vi "CCD photon image_Shaowei-v2.vi"() -> ()   [LabVIEW 2009]
uses:
  <vilib>/Utility/file.llb/Read From Spreadsheet File (DBL).vi
  Instance           5 35Saved   CCD photon image_540_800_CR .vi
  Instance           4 35Saved   CCD photon image_540_800_CR .vi
  Instance           3 35Saved   CCD photon image_540_800_CR .vi
  Instance           8 35Saved   CCD photon image_540_800_CR .vi
  <vilib>/Analysis/Matrix/Numeric/Conversions/Array To Matrix - RA2.vi
  Instance          12 35Saved   CCD photon image_540_800_CR .vi
  Instance          18 35Saved   CCD photon image_540_800_CR .vi
  <vilib>/Analysis/Matrix/NI_Matrix.lvlib
panel:
  in  "Save Matrix6":bool
  in  "Save Matrix5":bool
  in  "Save Matrix3":bool
  in  "Save Matrix4":bool
  out "Matrix 2":string
  in  "Save Matrix2":bool
  out "Matrix 1":string
  in  "Save Matrix1":bool
  in  "select 2":bool
  in  "select":bool
  in  "next 2":bool
  in  "next":bool
  in  "previous 2":bool
  in  "previous":bool
  in  "?":bool
  out "?":path
  out "?":path
  out "?":i32
  in  "?":bool
  in  "stop 2":bool
  in  "#6":bool
  in  "#5":bool
  in  "to":dbl=950.0
  in  "From":dbl=550.0
  out "Intensity Graph 6":dbl[][](graph)
  out "Col":dbl
  out "to":dbl
  out "Matrix 6":string
  in  "lstart (nm)":dbl
  in  "lend (nm)":dbl
  out "eV":dbl
  out "eV":dbl
  out "Intensity Graph 5":dbl[][](graph)
  out "Col":dbl
  out "to":dbl
  out "Matrix 5":string
  in  "lstart (nm)":dbl
  in  "lend (nm)":dbl
  out "eV":dbl
  out "eV":dbl
  in  "?":bool
  out "MAX":dbl
  out "MIN":dbl
  out "X":sgl
  out "Y":sgl
  out "to":dbl
  out "Col":dbl
  out "eV":dbl
  out "eV":dbl
  in  "lend (nm)":dbl
  in  "lstart (nm)":dbl
  out "eV":dbl
  out "eV":dbl
  in  "lend (nm)":dbl
  in  "lstart (nm)":dbl
  out "to":dbl
  out "Col":dbl
  out "to":dbl
  out "Col":dbl
  out "eV":dbl
  out "eV":dbl
  in  "lend (nm)":dbl
  in  "lstart (nm)":dbl
  in  "?":dbl=32.0
  out "eV":dbl
  out "eV":dbl
  in  "lend (nm)":dbl
  in  "lstart (nm)":dbl
  out "to":dbl
  out "Col":dbl
  in  "#3":bool
  in  "#4":bool
  in  "#2":bool
  out "Intensity Graph 4":dbl[][](graph)
  out "Matrix 4":string
  out "Intensity Graph 3":dbl[][](graph)
  out "Matrix 3":string
  out "Intensity Graph 2":dbl[][](graph)
  out "Intensity Graph":dbl[][](graph)
  # "Input File"
  # "2 Files"
  # "1 File"
  # "1st"
  # "2nd"
  # "Spectra Range"
  # "nm"
  # "nm"
  # "# of Pixel"
  # "Image Size"
  # "Bit"
  # "Active Matrix"
  # "ON"
  # "OFF"
  # "Cosmic Ray Removal"
  # "NO"
  # "YES"
  # "Value"
  # "Position"
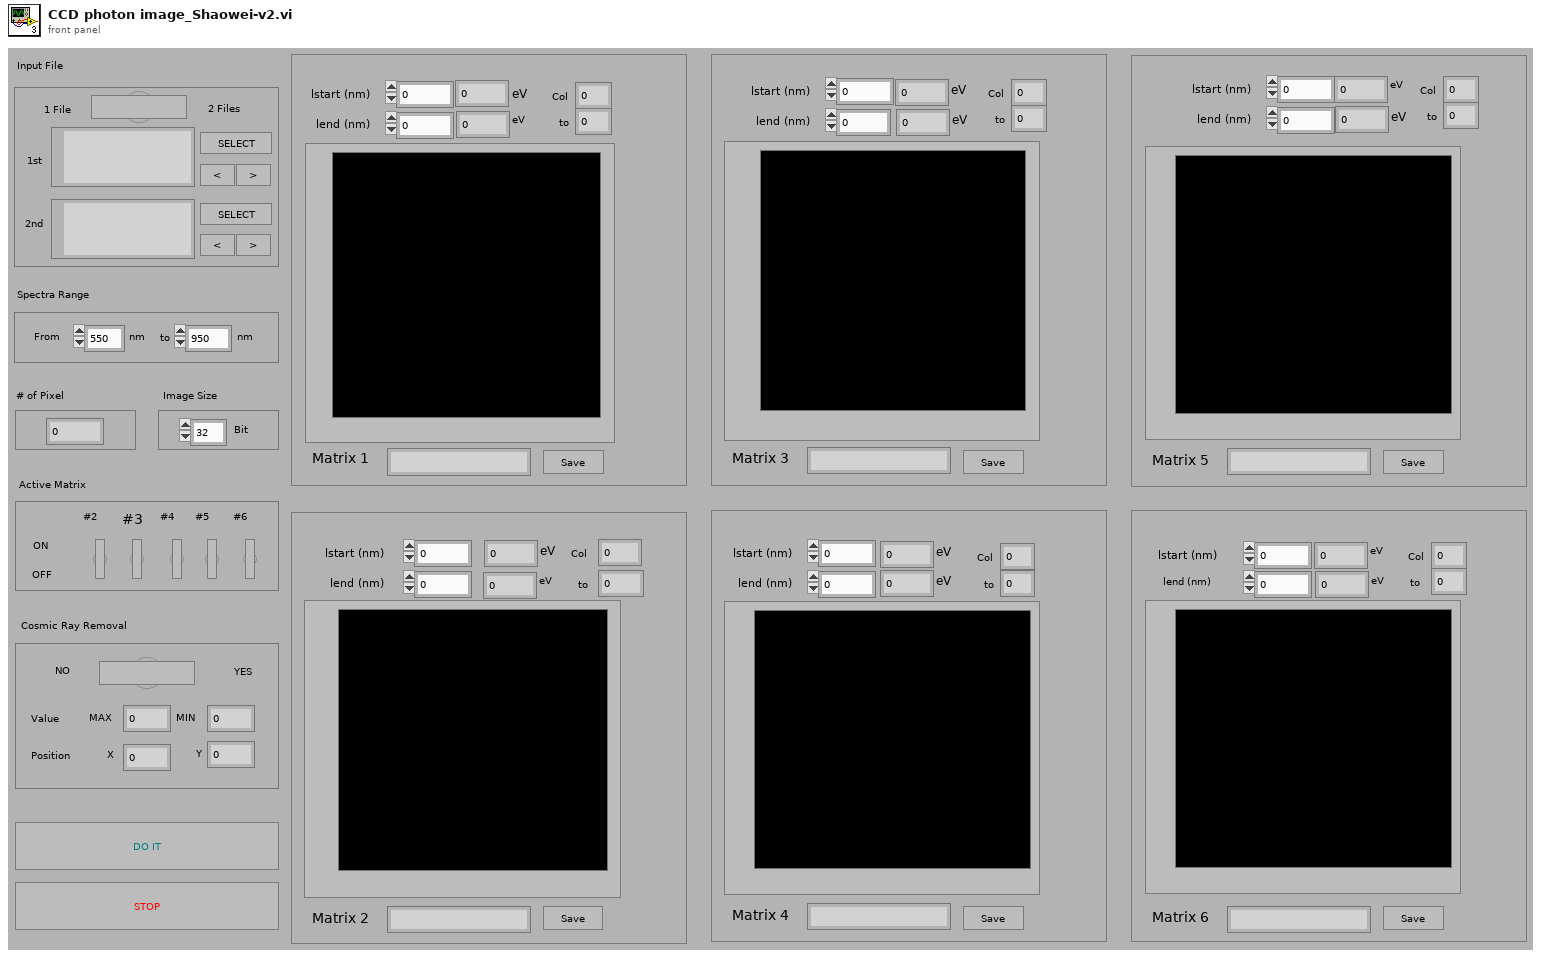
[diagram p1: front panel]
types:
  T1 = typedef "NI_Matrix.lvlib/RealMatrix.ctl" = dbl[][]
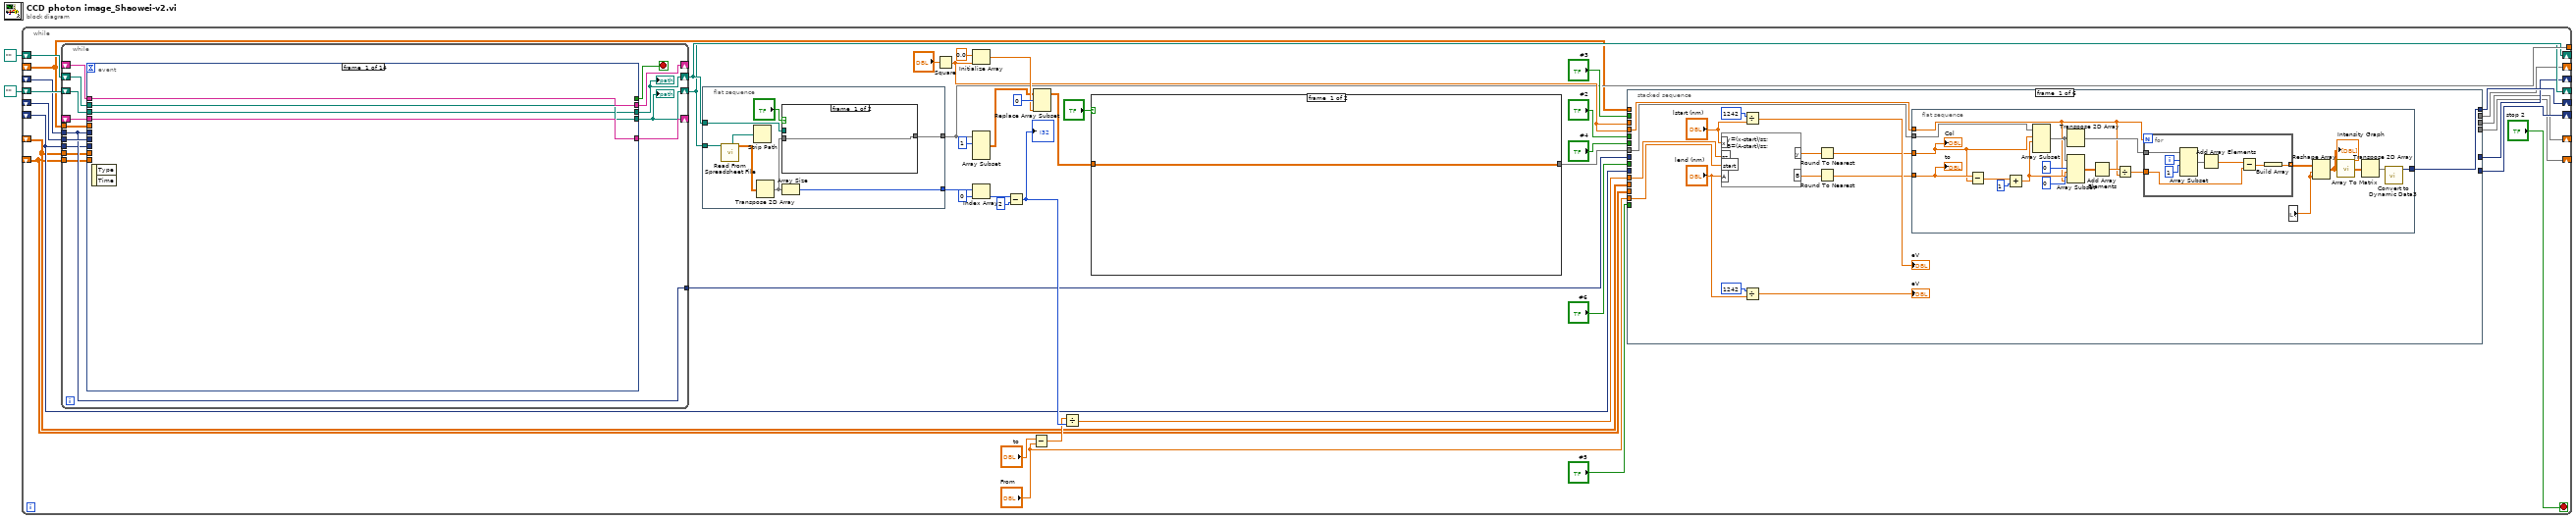
[diagram p0: block diagram]
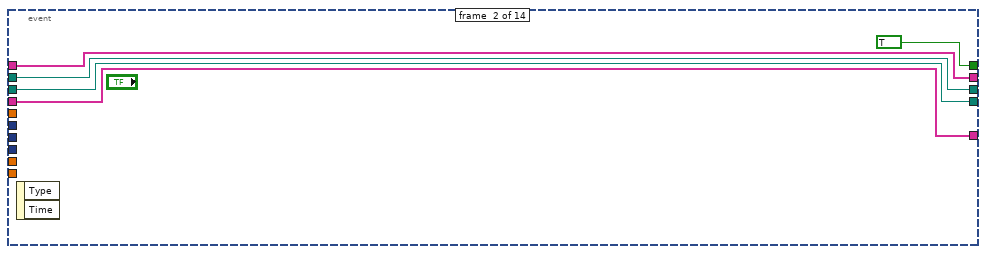
[diagram p2: hidden frame]
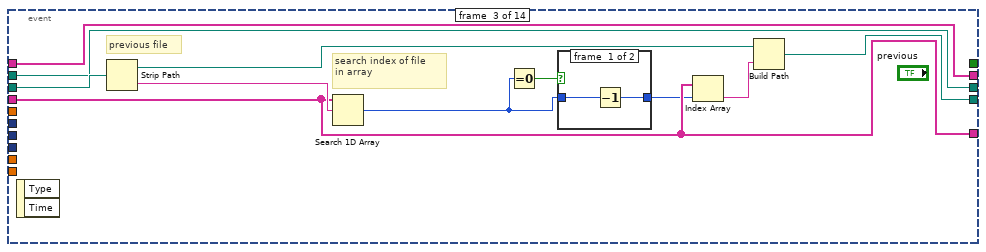
[diagram p3: hidden frame]
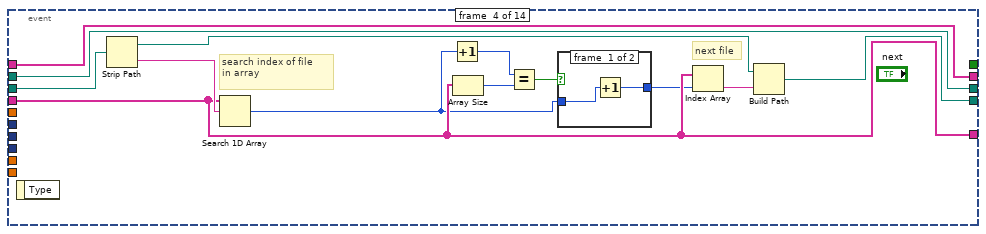
[diagram p5: hidden frame]
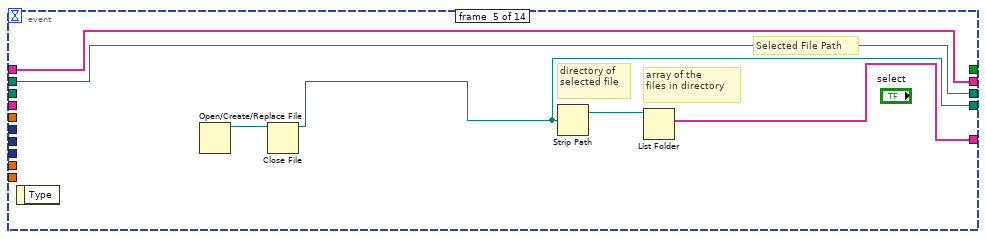
[diagram p7: hidden frame]
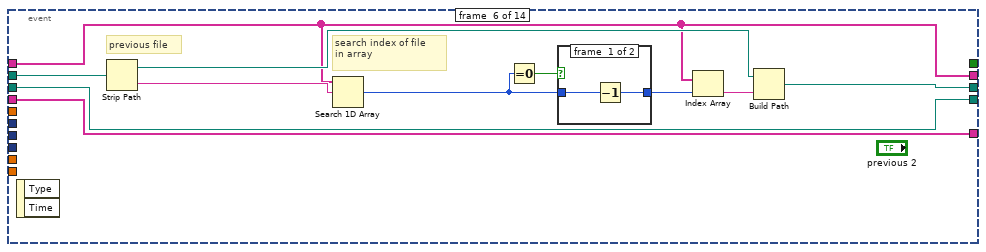
[diagram p8: hidden frame]
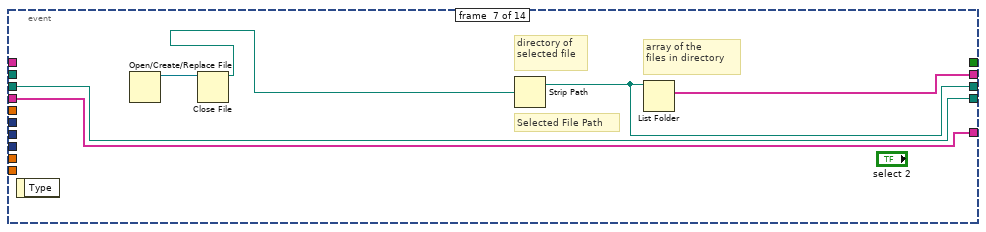
[diagram p10: hidden frame]
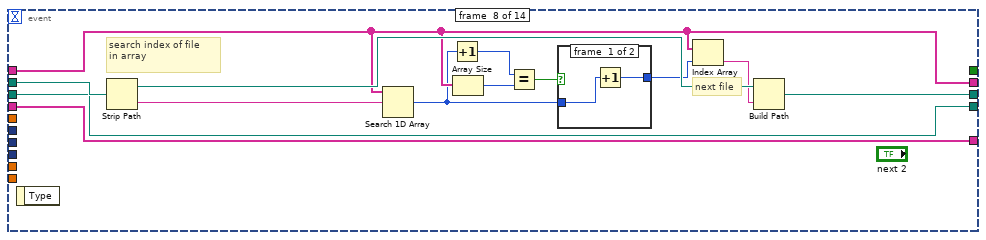
[diagram p11: hidden frame]
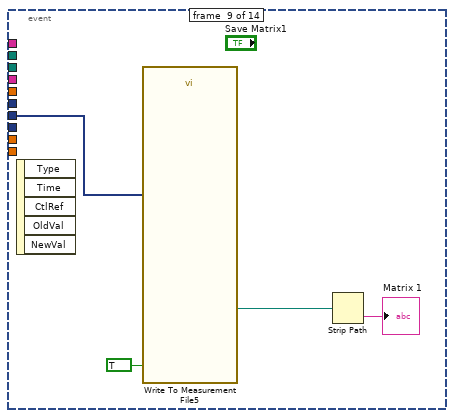
[diagram p13: hidden frame]
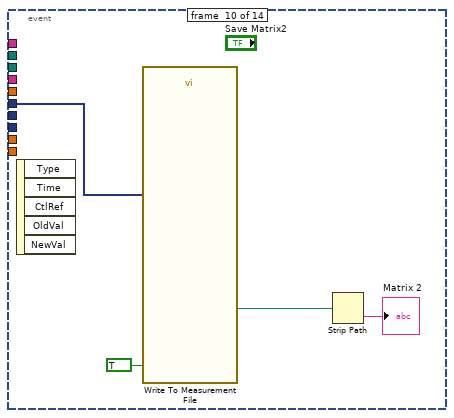
[diagram p14: hidden frame]
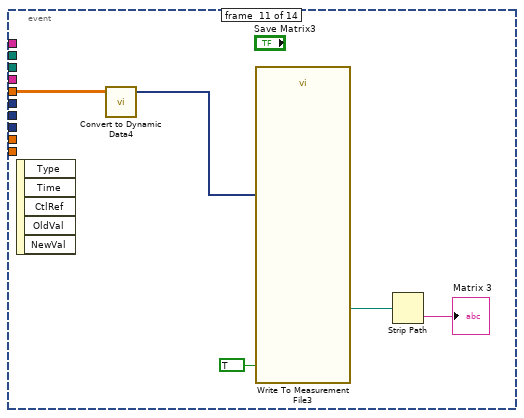
[diagram p15: hidden frame]
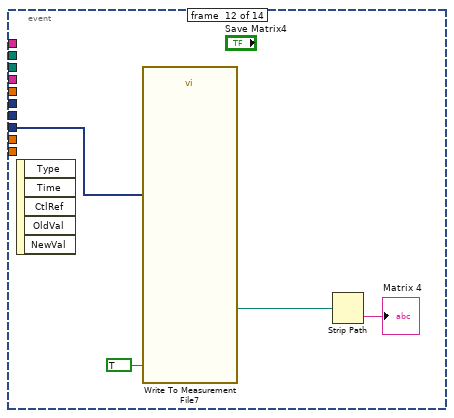
[diagram p16: hidden frame]
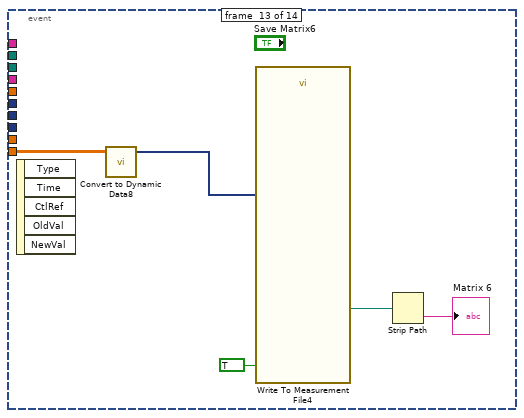
[diagram p17: hidden frame]
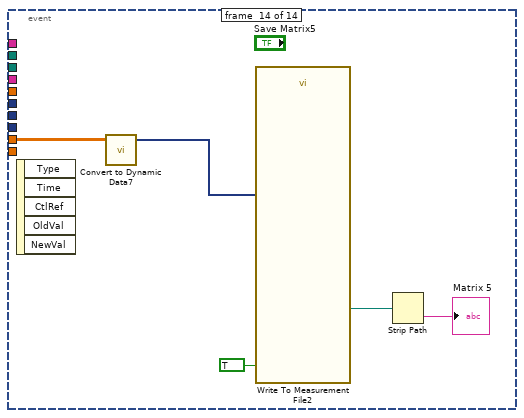
[diagram p18: hidden frame]
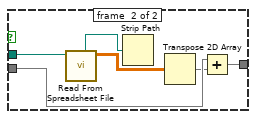
[diagram p19: hidden frame]
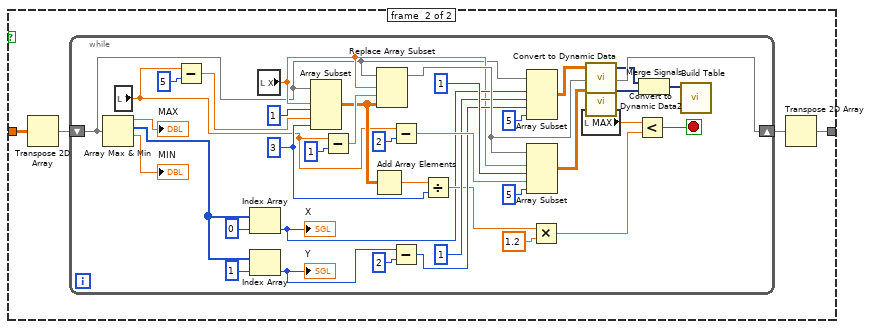
[diagram p20: hidden frame]
diagram:
  n1 = while {
    tunnel: [w26] -> _
    shift-right: [w16] -> _
    shift-left: path "" ("path") -> [w18]
    shift-right: [w17] -> _
    shift-left: path "" ("path") -> [w19]
    shift-right: [w15] -> _
    shift-left: _ -> [w14]
    shift-right: [w13] -> _
    shift-left: _ -> [w12]
    shift-right: [w10] -> _
    shift-left: _ -> [w9]
    shift-right: [w8] -> _
    shift-left: _ -> [w7]
    shift-right: [w6] -> _
    shift-left: _ -> [w5]
    shift-right: [w4] -> _
    shift-left: _ -> [w3]
    stop <- "stop 2" stop-if-true
    n2 = while {
      shift-right: [w60] -> _
      shift-left: _ -> [w59]
      shift-right: [w46] -> w16
      shift-left: w18 -> [w58]
      shift-right: [w47] -> w17
      shift-left: w19 -> [w57]
      shift-right: [w56] -> _
      shift-left: _ -> [w55]
      tunnel: w14 -> [w53]
      tunnel: w12 -> [w52]
      tunnel: [w52] -> w11
      tunnel: w9 -> [w51]
      tunnel: w7 -> [w50]
      tunnel: w5 -> [w49]
      tunnel: w3 -> [w48]
      stop <- w54 stop-if-true
      n3 = event shown="[4] \"select\": Value Change" {
        selector: _ -> [_ _ _ _ _ _ _ _ _ _ _ _ _ _]
        dyn-events: _ -> [_ _ _ _ _ _ _ _ _ _ _ _ _ _]
        timeout: _ -> [_ _ _ _ _ _ _ _ _ _ _ _ _ _]
        tunnel: [_ TRUE _ _ _ _ _ _ _ _ _ _ _ _] -> w54
        tunnel: [w63 w67 w75 w93 w100 w106 w124 w133 _ _ _ _ _ _] -> w46
        tunnel: [w64 w68 w77 w89 w104 w111 w123 w132 _ _ _ _ _ _] -> w60
        tunnel: w59 -> [w64 w68 w77 w89 _ w111 w123 w132 _ _ _ _ _ _]
        tunnel: w58 -> [w63 w67 w80 w92 _ w106 w124 w133 _ _ _ _ _ _]
        tunnel: [w61 w65 w73 w90 w102 w107 w122 w134 _ _ _ _ _ _] -> w47
        tunnel: w57 -> [w61 w65 w73 w90 w102 w113 _ w135 _ _ _ _ _ _]
        tunnel: [w62 w66 w74 w91 w103 w112 w125 w128 _ _ _ _ _ _] -> w56
        tunnel: w55 -> [w62 w66 w74 w91 w103 w112 _ w128 _ _ _ _ _ _]
        tunnel: w53 -> [_ _ _ _ _ _ _ _ w145 _ _ _ _ _]
        tunnel: w52 -> [_ _ _ _ _ _ _ _ _ w149 _ _ _ _]
        tunnel: w51 -> [_ _ _ _ _ _ _ _ _ _ _ w155 _ _]
        tunnel: w50 -> [_ _ _ _ _ _ _ _ _ _ w151 _ _ _]
        tunnel: w49 -> [_ _ _ _ _ _ _ _ _ _ _ _ _ w166]
        tunnel: w48 -> [_ _ _ _ _ _ _ _ _ _ _ _ w160 _]
        event #0 {
          n4 = event-data() -> ()  [unwired: 1 in, 2 out]
        }
        event #1 {
          n5 = event-data() -> ()  [unwired: 1 in, 2 out]
        }
        event #2 {
          # "previous file"
          # "search index of file\nin array"
          n6 = event-data() -> ()  [unwired: 1 in, 2 out]
          n7 = Strip Path(path=w80) -> (stripped path=w78:path, name=w79:string)
          n8 = Search 1D Array(1D array=w77, element=w79) -> (index of element=w71:i32)  [unwired: 1 in]
          n9 = Equal To 0?(x=w71) -> (x = 0?=w72:bool)
          n10 = case shown="False" w72 {
            tunnel: w71 -> [w82 w83]
            tunnel: [w81 w83] -> w70
            frame #0 {
              n11 = Decrement(x=w82) -> (x-1=w81:i32)
            }
            frame #1 {
            }
          }
          n12 = Index Array(array=w77, index=w70) -> (element=w76:string)
          n13 = Build Path(base path=w78, name or relative path=w76) -> (appended path=w75:path)
        }
        event #3 {
          # "next file"
          # "search index of file\nin array"
          n14 = event-data() -> ()  [unwired: 1 in, 1 out]
          n15 = Strip Path(path=w92) -> (stripped path=w95:path, name=w96:string)
          n16 = Search 1D Array(1D array=w89, element=w96) -> (index of element=w84:i32)  [unwired: 1 in]
          n17 = Increment(x=w84) -> (x+1=w85:i32)
          n18 = Array Size(array=w89) -> (size(s)=w88:i32)
          n19 = Equal?(x=w85, y=w88) -> (x = y?=w87:bool)
          n20 = case shown="True" w87 {
            tunnel: w84 -> [w98 w99]
            tunnel: [w97 w99] -> w86
            frame #0 {
              n21 = Increment(x=w98) -> (x+1=w97:i32)
            }
            frame #1 {
            }
          }
          n22 = Index Array(array=w89, index=w86) -> (element=w94:string)
          n23 = Build Path(base path=w95, name or relative path=w94) -> (appended path=w93:path)
        }
        event #4 {
          # "array of the \nfiles in directory"
          # "directory of\nselected file"
          # "Selected File Path"
          n24 = event-data() -> ()  [unwired: 1 in, 1 out]
          n25 = Open/Create/Replace File() -> (refnum out=w101:refnum<file>)  [unwired: 6 in, 2 out]
          n26 = Close File(refnum=w101) -> (path=w100:path)  [unwired: 1 in, 1 out]
          n27 = Strip Path(path=w100) -> (stripped path=w105:path)  [unwired: 1 out]
          n28 = List Folder(path=w105) -> (filenames=w104:string[])  [unwired: 3 in, 3 out]
        }
        event #5 {
          # "previous file"
          # "search index of file\nin array"
          n29 = event-data() -> ()  [unwired: 1 in, 2 out]
          n30 = Strip Path(path=w113) -> (stripped path=w115:path, name=w116:string)
          n31 = Search 1D Array(1D array=w112, element=w116) -> (index of element=w109:i32)  [unwired: 1 in]
          n32 = Equal To 0?(x=w109) -> (x = 0?=w110:bool)
          n33 = case shown="False" w110 {
            tunnel: w109 -> [w118 w119]
            tunnel: [w117 w119] -> w108
            frame #0 {
              n34 = Decrement(x=w118) -> (x-1=w117:i32)
            }
            frame #1 {
            }
          }
          n35 = Index Array(array=w112, index=w108) -> (element=w114:string)
          n36 = Build Path(base path=w115, name or relative path=w114) -> (appended path=w107:path)
        }
        event #6 {
          # "array of the \nfiles in directory"
          # "directory of\nselected file"
          # "Selected File Path"
          n37 = event-data() -> ()  [unwired: 1 in, 1 out]
          n38 = Open/Create/Replace File() -> (refnum out=w121:refnum<file>)  [unwired: 6 in, 2 out]
          n39 = Close File(refnum=w121) -> (path=w120:path)  [unwired: 1 in, 1 out]
          n40 = Strip Path(path=w120) -> (stripped path=w122:path)  [unwired: 1 out]
          n41 = List Folder(path=w122) -> (filenames=w125:string[])  [unwired: 3 in, 3 out]
        }
        event #7 {
          # "next file"
          # "search index of file\nin array"
          n42 = event-data() -> ()  [unwired: 1 in, 1 out]
          n43 = Strip Path(path=w135) -> (stripped path=w137:path, name=w138:string)
          n44 = Search 1D Array(1D array=w128, element=w138) -> (index of element=w127:i32)  [unwired: 1 in]
          n45 = Increment(x=w127) -> (x+1=w129:i32)
          n46 = Array Size(array=w128) -> (size(s)=w131:i32)
          n47 = Equal?(x=w129, y=w131) -> (x = y?=w130:bool)
          n48 = case shown="True" w130 {
            tunnel: w127 -> [w140 w141]
            tunnel: [w139 w141] -> w126
            frame #0 {
              n49 = Increment(x=w140) -> (x+1=w139:i32)
            }
            frame #1 {
            }
          }
          n50 = Index Array(array=w128, index=w126) -> (element=w136:string)
          n51 = Build Path(base path=w137, name or relative path=w136) -> (appended path=w134:path)
        }
        event #8 {
          n52 = event-data() -> ()  [unwired: 1 in, 5 out]
          n53 = call "Write To Measurement File5"("Signals"=w145, "Reset"=TRUE) -> ("Filename Out"=w143:path)  [unwired: 15 in, 2 out]
          n54 = Strip Path(path=w143) -> (name=→"Matrix 1":string)  [unwired: 1 out]
        }
        event #9 {
          n55 = event-data() -> ()  [unwired: 1 in, 5 out]
          n56 = call "Write To Measurement File"("Signals"=w149, "Reset"=TRUE) -> ("Filename Out"=w147:path)  [unwired: 15 in, 2 out]
          n57 = Strip Path(path=w147) -> (name=→"Matrix 2":string)  [unwired: 1 out]
        }
        event #10 {
          n58 = event-data() -> ()  [unwired: 1 in, 5 out]
          n59 = call "Convert to Dynamic Data4"("2D Array"=w151) -> ("Dynamic Data Type"=w150:dynamicdata)  [unwired: 3 in]
          n60 = call "Write To Measurement File3"("Signals"=w150, "Reset"=TRUE) -> ("Filename Out"=w154:path)  [unwired: 15 in, 2 out]
          n61 = Strip Path(path=w154) -> (name=→"Matrix 3":string)  [unwired: 1 out]
        }
        event #11 {
          n62 = event-data() -> ()  [unwired: 1 in, 5 out]
          n63 = call "Write To Measurement File7"("Signals"=w155, "Reset"=TRUE) -> ("Filename Out"=w157:path)  [unwired: 15 in, 2 out]
          n64 = Strip Path(path=w157) -> (name=→"Matrix 4":string)  [unwired: 1 out]
        }
        event #12 {
          n65 = event-data() -> ()  [unwired: 1 in, 5 out]
          n66 = call "Convert to Dynamic Data8"("2D Array"=w160) -> ("Dynamic Data Type"=w159:dynamicdata)  [unwired: 3 in]
          n67 = call "Write To Measurement File4"("Signals"=w159, "Reset"=TRUE) -> ("Filename Out"=w162:path)  [unwired: 15 in, 2 out]
          n68 = Strip Path(path=w162) -> (name=→"Matrix 6":string)  [unwired: 1 out]
        }
        event #13 {
          n69 = event-data() -> ()  [unwired: 1 in, 5 out]
          n70 = call "Convert to Dynamic Data7"("2D Array"=w166) -> ("Dynamic Data Type"=w165:dynamicdata)  [unwired: 3 in]
          n71 = call "Write To Measurement File2"("Signals"=w165, "Reset"=TRUE) -> ("Filename Out"=w167:path)  [unwired: 15 in, 2 out]
          n72 = Strip Path(path=w167) -> (name=→"Matrix 5":string)  [unwired: 1 out]
        }
      }
      "?" <- w46
      "?" <- w47
    }
    n73 = flat-sequence {
      tunnel: [w175] -> w26
      tunnel: [w172] -> w23
      tunnel: w16 -> [w170]
      tunnel: w17 -> [w169]
      frame #0 {
        n74 = call-poly <vilib>:"Read From Spreadsheet File.vi"("file path (dialog if empty)"=w170) -> ("all rows"=w173:dbl[][], "new file path (Not A Path if cancelled)"=w176:path)  [unwired: 6 in, 3 out]
        n75 = Strip Path(path=w176) -> ()  [unwired: 2 out]
        n76 = Transpose 2D Array(2D array=w173) -> (transposed array=w171:dbl[][])
        n77 = case shown="False" "?" {
          tunnel: w171 -> [w177 w182]
          tunnel: [w177 w181] -> w175
          tunnel: w169 -> [_ w178]
          frame #0 {
          }
          frame #1 {
            n78 = call-poly <vilib>:"Read From Spreadsheet File.vi"("file path (dialog if empty)"=w178) -> ("all rows"=w180:dbl[][], "new file path (Not A Path if cancelled)"=w183:path)  [unwired: 6 in, 3 out]
            n79 = Strip Path(path=w183) -> ()  [unwired: 2 out]
            n80 = Transpose 2D Array(2D array=w180) -> (transposed array=w179:dbl[][])
            n81 = Add(x=w182, y=w179) -> (x+y=w181:dbl[][])
          }
        }
        n82 = Array Size(array=w171) -> (size(s)=w172:i32[])
      }
    }
    n83 = Square(x="?") -> (x^2=w37:dbl)
    n84 = Initialize Array(0.0 ("element"), w37) -> (w41:dbl[])
    n85 = Array Subset(array=w26, index (row)=1) -> (w39:dbl[][])  [unwired: 3 in]
    n86 = Index Array(array=w23, index=0) -> (element=w21:i32)
    n87 = Subtract(x=w21, y=2) -> (x-y=w33:i32)
    "?" <- w33
    n88 = Subtract(x="to", y="From") -> (x-y=w32:dbl)
    n89 = Replace Array Subset(array=w39, new element=w41, index (row)=0) -> (w36:dbl[][])  [unwired: 1 in]
    n90 = Divide(x=w32, y=w33) -> (x/y=w31:dbl)
    n91 = case shown="True" "?" {
      tunnel: w36 -> [w184 w188]
      tunnel: [w184 w186] -> w35
      frame #0 {
      }
      frame #1 {
        n92 = Transpose 2D Array(2D array=w188) -> (transposed array=w187:dbl[][])
        n93 = while {
          shift-right: [w225] -> w185
          shift-left: w187 -> [w189]
          stop <- w204 stop-if-true
          w202 = 3
          n94 = Array Max & Min(array=w189) -> (max value=→"MAX":dbl, max index (indices)=w223:i32[], min value=→"MIN":dbl)  [unwired: 1 out]
          n95 = local read "Y"() -> (w191:sgl)
          n96 = Subtract(x=w191, y=5) -> (x-y=w219:sgl)
          n97 = Index Array(array=w223, index=0) -> (element=w196:i32)
          "X" <- w196
          n98 = Index Array(array=w223, index=1) -> (element=w195:i32)
          "Y" <- w195
          n99 = local read "X"() -> (w192:sgl)
          n100 = Array Subset(array=w189, index (row)=w192, length (row)=1, index (col)=w219, length (col)=w202) -> (w201:dbl[][])
          n101 = Subtract(x=w191, y=1) -> (x-y=w218:sgl)
          n102 = Add Array Elements(numeric array=w201) -> (sum=w203:dbl)
          n103 = Replace Array Subset(array=w189, new element=w201, index (row)=w192, index (col)=w218) -> (w225:dbl[][])
          n104 = Subtract(x=w191, y=2) -> (x-y=w214:sgl)
          n105 = Subtract(x=w195, y=2) -> (x-y=w209:i32)
          n106 = Divide(x=w203, y=w202) -> (x/y=w200:dbl)
          n107 = Array Subset(array=w189, index (row)=w196, length (row)=1, index (col)=w209, length (col)=5) -> (w207:dbl[][])
          n108 = Array Subset(array=w225, index (row)=w192, length (row)=1, index (col)=w214, length (col)=5) -> (w212:dbl[][])
          n109 = Multiply(x=w200, y=1.2) -> (x*y=w205:dbl)
          n110 = local read "MAX"() -> (w190:dbl)
          n111 = call "Convert to Dynamic Data"("2D Array"=w207) -> ("Dynamic Data Type"=w199:dynamicdata)  [unwired: 3 in]
          n112 = call "Convert to Dynamic Data2"("2D Array"=w212) -> ("Dynamic Data Type"=w197:dynamicdata)  [unwired: 3 in]
          n113 = Less?(x=w190, y=w205) -> (x < y?=w204:bool)
          n114 = Merge Signals(w199, w197) -> (w198:dynamicdata)
          n115 = call "Build Table"("Signals"=w198) -> ()  [unwired: 9 in, 2 out]
        }
        n116 = Transpose 2D Array(2D array=w185) -> (transposed array=w186:dbl[][])
      }
    }
    n117 = stacked-sequence {
      tunnel: "#4" -> [_ _ _ w376 _ _]
      tunnel: "#3" -> [_ _ w326 _ _ _]
      tunnel: "#2" -> [_ w275 _ _ _ _]
      tunnel: w37 -> [w230 w274 w325 _ _ _]
      tunnel: w35 -> [w229 w273 w324 w374 w426 w476]
      tunnel: w37 -> [_ _ _ w375 w427 w477]
      tunnel: w31 -> [w228 w272 w323 w372 w425 w475]
      tunnel: "From" -> [w227 w271 w322 w373 w424 w474]
      tunnel: "#5" -> [_ _ _ _ w423 _]
      tunnel: "#6" -> [_ _ _ _ _ w473]
      tunnel: [w226 _ _ _ _ _] -> w15
      tunnel: [_ w270 _ _ _ _] -> w13
      tunnel: w11 -> [_ w269 _ _ _ _]
      tunnel: [_ _ _ w371 _ _] -> w10
      tunnel: w9 -> [_ _ _ w370 _ _]
      tunnel: [_ _ w321 _ _ _] -> w8
      tunnel: w7 -> [_ _ w320 _ _ _]
      tunnel: [_ _ _ _ w422 _] -> w6
      tunnel: w5 -> [_ _ _ _ w421 _]
      tunnel: [_ _ _ _ _ w472] -> w4
      tunnel: w3 -> [_ _ _ _ _ w471]
      frame #0 {
        n118 = formula code="y=(x-start)/sz;\nB=(A-start)/sz;"("x"="lstart (nm)", "A"="lend (nm)", "sz"=w228, "start"=w227) -> ("y"=w234:dbl, "B"=w233:dbl)
        n119 = Divide(x=1242, y="lstart (nm)") -> (x/y=→"eV":dbl)
        n120 = Divide(x=1242, y="lend (nm)") -> (x/y=→"eV":dbl)
        n121 = Round To Nearest(number=w234) -> (nearest integer value=w232:dbl)
        n122 = Round To Nearest(number=w233) -> (nearest integer value=w231:dbl)
        n123 = flat-sequence {
          tunnel: [w260] -> w226
          tunnel: w231 -> [w253]
          tunnel: w232 -> [w252]
          tunnel: w230 -> [w241]
          tunnel: w229 -> [w245]
          frame #0 {
            n124 = Subtract(x=w253, y=w252) -> (x-y=w248:dbl)
            n125 = Add(x=w248, y=1) -> (x+y=w246:dbl)
            n126 = Array Subset(array=w245, index (row)=w252, length (row)=w246) -> (w244:dbl[][])  [unwired: 2 in]
            n127 = Transpose 2D Array(2D array=w244) -> (transposed array=w255:dbl[][])
            n128 = Array Subset(array=w244, index (row)=0, length (row)=w246, index (col)=0, length (col)=w241) -> (w243:dbl[][])
            n129 = Add Array Elements(numeric array=w243) -> (sum=w249:dbl)
            n130 = Divide(x=w249, y=w241) -> (x/y=w247:dbl)
            n131 = for {
              N: w241 -> [_]
              tunnel: w255 -> [w262]
              tunnel: [w264] -> w254 mode=indexing
              tunnel: w247 -> [w263]
              i -> [w268]
              n132 = Array Subset(array=w262, index (row)=w268, length (row)=1) -> (w261:dbl[][])  [unwired: 2 in]
              n133 = Add Array Elements(numeric array=w261) -> (sum=w266:dbl)
              n134 = Subtract(x=w266, y=w263) -> (x-y=w265:dbl)
              n135 = Build Array(w265) -> (w264:dbl[])
            }
            n136 = local read item#15() -> (w242:dbl)
            n137 = Reshape Array(w254, w242, w242) -> (w256:dbl[][])
            "Intensity Graph" <- w256
            n138 = call-poly <vilib>:"Array To Matrix.vi"("Real 2D Array"=w256) -> ("Real Matrix"=w259:T1)
            n139 = Transpose 2D Array(2D array=w259) -> (transposed array=w258:T1)
            n140 = call "Convert to Dynamic Data3"("2D Array"=w258) -> ("Dynamic Data Type"=w260:dynamicdata)  [unwired: 3 in]
            "Col" <- w252
            "to" <- w253
          }
        }
      }
      frame #1 {
        n141 = case shown="True" w275 {
          tunnel: w274 -> [_ w282]
          tunnel: w273 -> [_ w281]
          tunnel: w272 -> [_ w280]
          tunnel: w271 -> [_ w279]
          tunnel: [w276 w277] -> w270
          tunnel: w269 -> [w276 _]
          frame #0 {
          }
          frame #1 {
            n142 = formula code="y=(x-start)/sz;\nB=(A-start)/sz;"("x"="lstart (nm)", "A"="lend (nm)", "sz"=w280, "start"=w279) -> ("y"=w286:dbl, "B"=w285:dbl)
            n143 = Divide(x=1242, y="lend (nm)") -> (x/y=→"eV":dbl)
            n144 = Divide(x=1242, y="lstart (nm)") -> (x/y=→"eV":dbl)
            n145 = Round To Nearest(number=w286) -> (nearest integer value=w284:dbl)
            n146 = Round To Nearest(number=w285) -> (nearest integer value=w283:dbl)
            n147 = flat-sequence {
              tunnel: w284 -> [w298]
              tunnel: w283 -> [w299]
              tunnel: [w306] -> w278
              tunnel: w282 -> [w294]
              tunnel: w281 -> [w293]
              frame #0 {
                n148 = Subtract(x=w299, y=w298) -> (x-y=w307:dbl)
                n149 = Add(x=w307, y=1) -> (x+y=w301:dbl)
                n150 = Array Subset(array=w293, index (row)=w298, length (row)=w301) -> (w297:dbl[][])  [unwired: 2 in]
                n151 = Transpose 2D Array(2D array=w297) -> (transposed array=w310:dbl[][])
                n152 = Array Subset(array=w297, index (row)=0, length (row)=w301, index (col)=0, length (col)=w294) -> (w295:dbl[][])
                n153 = Add Array Elements(numeric array=w295) -> (sum=w304:dbl)
                n154 = Divide(x=w304, y=w294) -> (x/y=w300:dbl)
                n155 = for {
                  N: w294 -> [_]
                  tunnel: w310 -> [w319]
                  tunnel: [w312] -> w311 mode=indexing
                  tunnel: w300 -> [w314]
                  i -> [w318]
                  n156 = Array Subset(array=w319, index (row)=w318, length (row)=1) -> (w317:dbl[][])  [unwired: 2 in]
                  n157 = Add Array Elements(numeric array=w317) -> (sum=w315:dbl)
                  n158 = Subtract(x=w315, y=w314) -> (x-y=w313:dbl)
                  n159 = Build Array(w313) -> (w312:dbl[])
                }
                n160 = local read item#15() -> (w296:dbl)
                n161 = Reshape Array(w311, w296, w296) -> (w309:dbl[][])
                "Intensity Graph 2" <- w309
                n162 = call-poly <vilib>:"Array To Matrix.vi"("Real 2D Array"=w309) -> ("Real Matrix"=w305:T1)
                n163 = Transpose 2D Array(2D array=w305) -> (transposed array=w306:T1)
                "Col" <- w298
                "to" <- w299
              }
            }
            n164 = call "Convert to Dynamic Data5"("2D Array"=w278) -> ("Dynamic Data Type"=w277:dynamicdata)  [unwired: 3 in]
          }
        }
      }
      frame #2 {
        n165 = case shown="False" w326 {
          tunnel: w325 -> [_ w332]
          tunnel: w324 -> [_ w331]
          tunnel: w323 -> [_ w330]
          tunnel: w322 -> [_ w329]
          tunnel: [w327 w328] -> w321
          tunnel: w320 -> [w327 _]
          frame #0 {
          }
          frame #1 {
            n166 = formula code="y=(x-start)/sz;\nB=(A-start)/sz;"("x"="lstart (nm)", "A"="lend (nm)", "sz"=w330, "start"=w329) -> ("y"=w340:dbl, "B"=w339:dbl)
            n167 = Divide(x=1242, y="lstart (nm)") -> (x/y=→"eV":dbl)
            n168 = Divide(x=1242, y="lend (nm)") -> (x/y=→"eV":dbl)
            n169 = Round To Nearest(number=w340) -> (nearest integer value=w338:dbl)
            n170 = Round To Nearest(number=w339) -> (nearest integer value=w337:dbl)
            n171 = flat-sequence {
              tunnel: w337 -> [w348]
              tunnel: w338 -> [w349]
              tunnel: [w356] -> w328
              tunnel: w332 -> [w344]
              tunnel: w331 -> [w343]
              frame #0 {
                n172 = Subtract(x=w348, y=w349) -> (x-y=w357:dbl)
                n173 = Add(x=w357, y=1) -> (x+y=w351:dbl)
                n174 = Array Subset(array=w343, index (row)=w349, length (row)=w351) -> (w345:dbl[][])  [unwired: 2 in]
                n175 = Transpose 2D Array(2D array=w345) -> (transposed array=w360:dbl[][])
                n176 = Array Subset(array=w345, index (row)=0, length (row)=w351, index (col)=0, length (col)=w344) -> (w346:dbl[][])
                n177 = Add Array Elements(numeric array=w346) -> (sum=w352:dbl)
                n178 = Divide(x=w352, y=w344) -> (x/y=w350:dbl)
                n179 = for {
                  N: w344 -> [_]
                  tunnel: w360 -> [w369]
                  tunnel: [w363] -> w361 mode=indexing
                  tunnel: w350 -> [w362]
                  i -> [w368]
                  n180 = Array Subset(array=w369, index (row)=w368, length (row)=1) -> (w367:dbl[][])  [unwired: 2 in]
                  n181 = Add Array Elements(numeric array=w367) -> (sum=w365:dbl)
                  n182 = Subtract(x=w365, y=w362) -> (x-y=w364:dbl)
                  n183 = Build Array(w364) -> (w363:dbl[])
                }
                n184 = local read item#15() -> (w347:dbl)
                n185 = Reshape Array(w361, w347, w347) -> (w359:dbl[][])
                "Intensity Graph 3" <- w359
                n186 = call-poly <vilib>:"Array To Matrix.vi"("Real 2D Array"=w359) -> ("Real Matrix"=w355:T1)
                n187 = Transpose 2D Array(2D array=w355) -> (transposed array=w356:T1)
                "Col" <- w349
                "to" <- w348
              }
            }
          }
        }
      }
      frame #3 {
        n188 = case shown="False" w376 {
          tunnel: w375 -> [_ w383]
          tunnel: w374 -> [_ w382]
          tunnel: w373 -> [_ w381]
          tunnel: w372 -> [_ w380]
          tunnel: [w377 w378] -> w371
          tunnel: w370 -> [w377 _]
          frame #0 {
          }
          frame #1 {
            n189 = formula code="y=(x-start)/sz;\nB=(A-start)/sz;"("x"="lstart (nm)", "A"="lend (nm)", "sz"=w380, "start"=w381) -> ("y"=w391:dbl, "B"=w390:dbl)
            n190 = Divide(x=1242, y="lstart (nm)") -> (x/y=→"eV":dbl)
            n191 = Divide(x=1242, y="lend (nm)") -> (x/y=→"eV":dbl)
            n192 = Round To Nearest(number=w391) -> (nearest integer value=w385:dbl)
            n193 = Round To Nearest(number=w390) -> (nearest integer value=w384:dbl)
            n194 = flat-sequence {
              tunnel: w385 -> [w401]
              tunnel: w384 -> [w400]
              tunnel: [w408] -> w379
              tunnel: w383 -> [w394]
              tunnel: w382 -> [w395]
              frame #0 {
                n195 = Subtract(x=w400, y=w401) -> (x-y=w409:dbl)
                n196 = Add(x=w409, y=1) -> (x+y=w402:dbl)
                n197 = Array Subset(array=w395, index (row)=w401, length (row)=w402) -> (w399:dbl[][])  [unwired: 2 in]
                n198 = Transpose 2D Array(2D array=w399) -> (transposed array=w398:dbl[][])
                n199 = Array Subset(array=w399, index (row)=0, length (row)=w402, index (col)=0, length (col)=w394) -> (w396:dbl[][])
                n200 = Add Array Elements(numeric array=w396) -> (sum=w404:dbl)
                n201 = Divide(x=w404, y=w394) -> (x/y=w403:dbl)
                n202 = for {
                  N: w394 -> [_]
                  tunnel: w398 -> [w420]
                  tunnel: [w414] -> w412 mode=indexing
                  tunnel: w403 -> [w413]
                  i -> [w419]
                  n203 = Array Subset(array=w420, index (row)=w419, length (row)=1) -> (w418:dbl[][])  [unwired: 2 in]
                  n204 = Add Array Elements(numeric array=w418) -> (sum=w416:dbl)
                  n205 = Subtract(x=w416, y=w413) -> (x-y=w415:dbl)
                  n206 = Build Array(w415) -> (w414:dbl[])
                }
                n207 = local read item#15() -> (w397:dbl)
                n208 = Reshape Array(w412, w397, w397) -> (w411:dbl[][])
                "Intensity Graph 4" <- w411
                n209 = call-poly <vilib>:"Array To Matrix.vi"("Real 2D Array"=w411) -> ("Real Matrix"=w407:T1)
                n210 = Transpose 2D Array(2D array=w407) -> (transposed array=w408:T1)
                "Col" <- w401
                "to" <- w400
              }
            }
            n211 = call "Convert to Dynamic Data6"("2D Array"=w379) -> ("Dynamic Data Type"=w378:dynamicdata)  [unwired: 3 in]
          }
        }
      }
      frame #4 {
        n212 = case shown="False" w423 {
          tunnel: w427 -> [_ w433]
          tunnel: w426 -> [_ w432]
          tunnel: w425 -> [_ w431]
          tunnel: w424 -> [_ w430]
          tunnel: [w428 w429] -> w422
          tunnel: w421 -> [w428 _]
          frame #0 {
          }
          frame #1 {
            n213 = formula code="y=(x-start)/sz;\nB=(A-start)/sz;"("x"="lstart (nm)", "A"="lend (nm)", "sz"=w431, "start"=w430) -> ("y"=w441:dbl, "B"=w440:dbl)
            n214 = Divide(x=1242, y="lstart (nm)") -> (x/y=→"eV":dbl)
            n215 = Divide(x=1242, y="lend (nm)") -> (x/y=→"eV":dbl)
            n216 = Round To Nearest(number=w441) -> (nearest integer value=w435:dbl)
            n217 = Round To Nearest(number=w440) -> (nearest integer value=w434:dbl)
            n218 = flat-sequence {
              tunnel: w435 -> [w451]
              tunnel: w434 -> [w450]
              tunnel: [w458] -> w429
              tunnel: w433 -> [w444]
              tunnel: w432 -> [w445]
              frame #0 {
                n219 = Subtract(x=w450, y=w451) -> (x-y=w459:dbl)
                n220 = Add(x=w459, y=1) -> (x+y=w452:dbl)
                n221 = Array Subset(array=w445, index (row)=w451, length (row)=w452) -> (w449:dbl[][])  [unwired: 2 in]
                n222 = Transpose 2D Array(2D array=w449) -> (transposed array=w448:dbl[][])
                n223 = Array Subset(array=w449, index (row)=0, length (row)=w452, index (col)=0, length (col)=w444) -> (w446:dbl[][])
                n224 = Add Array Elements(numeric array=w446) -> (sum=w454:dbl)
                n225 = Divide(x=w454, y=w444) -> (x/y=w453:dbl)
                n226 = for {
                  N: w444 -> [_]
                  tunnel: w448 -> [w470]
                  tunnel: [w464] -> w462 mode=indexing
                  tunnel: w453 -> [w463]
                  i -> [w469]
                  n227 = Array Subset(array=w470, index (row)=w469, length (row)=1) -> (w468:dbl[][])  [unwired: 2 in]
                  n228 = Add Array Elements(numeric array=w468) -> (sum=w466:dbl)
                  n229 = Subtract(x=w466, y=w463) -> (x-y=w465:dbl)
                  n230 = Build Array(w465) -> (w464:dbl[])
                }
                n231 = local read item#15() -> (w447:dbl)
                n232 = Reshape Array(w462, w447, w447) -> (w461:dbl[][])
                "Intensity Graph 5" <- w461
                n233 = call-poly <vilib>:"Array To Matrix.vi"("Real 2D Array"=w461) -> ("Real Matrix"=w457:T1)
                n234 = Transpose 2D Array(2D array=w457) -> (transposed array=w458:T1)
                "Col" <- w451
                "to" <- w450
              }
            }
          }
        }
      }
      frame #5 {
        n235 = case shown="False" w473 {
          tunnel: w477 -> [_ w483]
          tunnel: w476 -> [_ w482]
          tunnel: w475 -> [_ w481]
          tunnel: w474 -> [_ w480]
          tunnel: [w478 w479] -> w472
          tunnel: w471 -> [w478 _]
          frame #0 {
          }
          frame #1 {
            n236 = formula code="y=(x-start)/sz;\nB=(A-start)/sz;"("x"="lstart (nm)", "A"="lend (nm)", "sz"=w481, "start"=w480) -> ("y"=w491:dbl, "B"=w490:dbl)
            n237 = Divide(x=1242, y="lstart (nm)") -> (x/y=→"eV":dbl)
            n238 = Divide(x=1242, y="lend (nm)") -> (x/y=→"eV":dbl)
            n239 = Round To Nearest(number=w491) -> (nearest integer value=w485:dbl)
            n240 = Round To Nearest(number=w490) -> (nearest integer value=w484:dbl)
            n241 = flat-sequence {
              tunnel: w485 -> [w501]
              tunnel: w484 -> [w500]
              tunnel: [w508] -> w479
              tunnel: w483 -> [w494]
              tunnel: w482 -> [w495]
              frame #0 {
                n242 = Subtract(x=w500, y=w501) -> (x-y=w509:dbl)
                n243 = Add(x=w509, y=1) -> (x+y=w502:dbl)
                n244 = Array Subset(array=w495, index (row)=w501, length (row)=w502) -> (w499:dbl[][])  [unwired: 2 in]
                n245 = Transpose 2D Array(2D array=w499) -> (transposed array=w498:dbl[][])
                n246 = Array Subset(array=w499, index (row)=0, length (row)=w502, index (col)=0, length (col)=w494) -> (w496:dbl[][])
                n247 = Add Array Elements(numeric array=w496) -> (sum=w504:dbl)
                n248 = Divide(x=w504, y=w494) -> (x/y=w503:dbl)
                n249 = for {
                  N: w494 -> [_]
                  tunnel: w498 -> [w520]
                  tunnel: [w514] -> w512 mode=indexing
                  tunnel: w503 -> [w513]
                  i -> [w519]
                  n250 = Array Subset(array=w520, index (row)=w519, length (row)=1) -> (w518:dbl[][])  [unwired: 2 in]
                  n251 = Add Array Elements(numeric array=w518) -> (sum=w516:dbl)
                  n252 = Subtract(x=w516, y=w513) -> (x-y=w515:dbl)
                  n253 = Build Array(w515) -> (w514:dbl[])
                }
                n254 = local read item#15() -> (w497:dbl)
                n255 = Reshape Array(w512, w497, w497) -> (w511:dbl[][])
                "Intensity Graph 6" <- w511
                n256 = call-poly <vilib>:"Array To Matrix.vi"("Real 2D Array"=w511) -> ("Real Matrix"=w507:T1)
                n257 = Transpose 2D Array(2D array=w507) -> (transposed array=w508:T1)
                "Col" <- w501
                "to" <- w500
              }
            }
          }
        }
      }
    }
  }
